vi "Create Network Message.vi"(6 "Remote Process":string, 7 "Remote IP":string, 9 "Value":string, 10 "Name":string, 11 "Message queue":refnum<queue>) -> (2 "Message":T1, 3 "Message queue out":refnum<queue>)   [LabVIEW 2021]
uses:
  Message.ctl
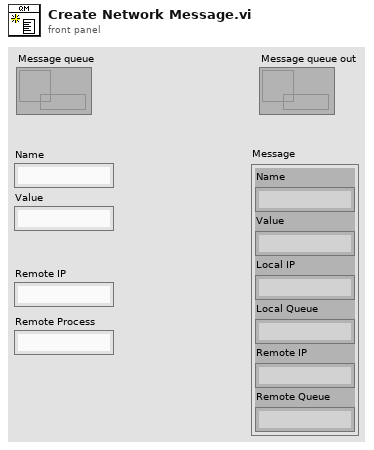
[diagram p1: front panel]
types:
  T1 = typedef "Message.ctl" = cluster{"Name":string, "Value":string, "Local IP":string, "Local Queue":string, "Remote IP":string, "Remote Queue":string}
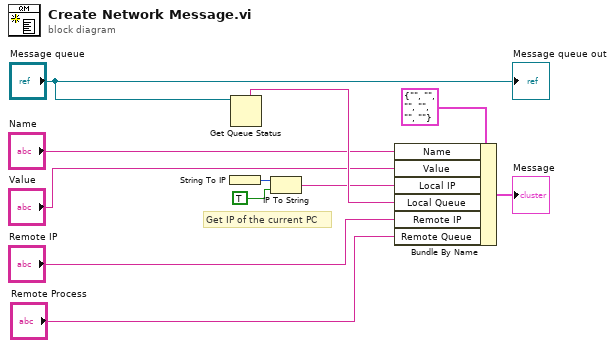
[diagram p0: block diagram]
diagram:
  # "Get IP of the current PC"
  n1 = String To IP() -> (0:w9:u32)  [unwired: 1 in]
  n2 = Get Queue Status(queue="Message queue") -> (queue name=w10:string)  [unwired: 2 in, 7 out]
  n3 = IP To String(1:TRUE ("dot notation? (F)"), 2:w9) -> (0:w8:string)
  n4 = Bundle By Name(cluster=T1 {"Name"="", "Value"="", "Local IP"="", "Local Queue"="", "Remote IP"="", "Remote Queue"=""} ("Message"), "Name"="Name", "Value"="Value", "Local IP"=w8, "Local Queue"=w10, "Remote IP"="Remote IP", "Remote Queue"="Remote Process") -> (→"Message":T1)
  "Message queue out" <- "Message queue"
